vi "GetRelativeAngle.vi"(8 "error in (no error)":errorcluster, 10 "Boat Angle":dbl, 11 "Angle in":refnum<class "Angle.lvclass">) -> (0 "error out":errorcluster, 2 "Relative Angle":dbl)   [LabVIEW 2011, in "Angle.lvclass"]
uses:
  Angle.lvclass
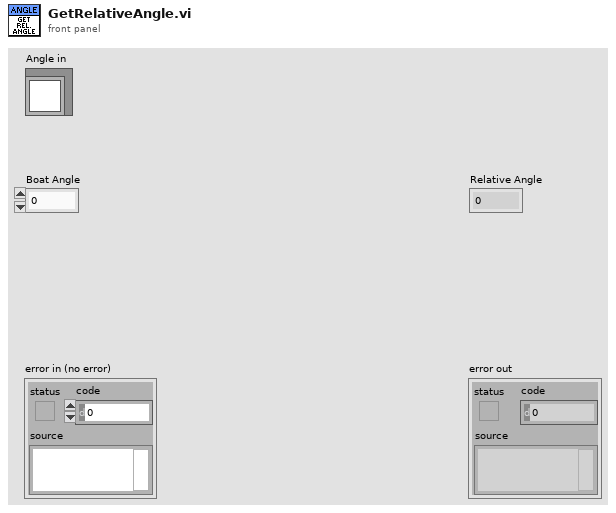
[diagram p1: front panel]
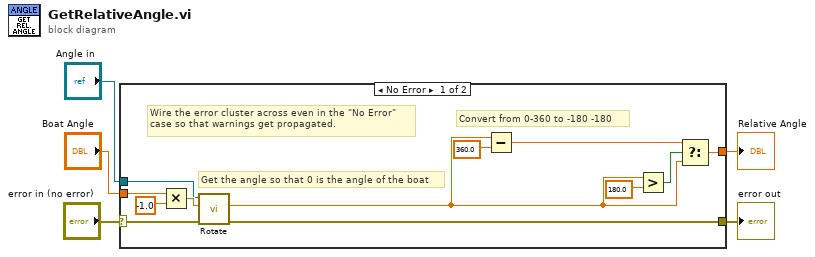
[diagram p0: block diagram]
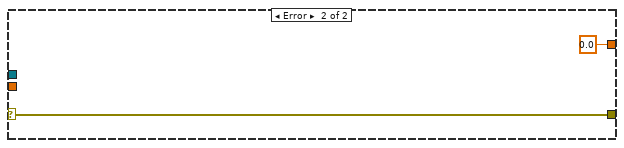
[diagram p2: hidden frame]
diagram:
  n1 = case shown="No Error" "error in (no error)" {
    selector: "error in (no error)" -> [w17 w19]
    tunnel: [w16 w19] -> w4
    tunnel: "Angle in" -> [w12 _]
    tunnel: "Boat Angle" -> [w14 _]
    tunnel: [w6 0.0 ("New Angle")] -> w1
    frame No Error {
      # "Convert from 0-360 to -180 -180"
      # "Get the angle so that 0 is the angle of the boat"
      # "Wire the error cluster across even in the \"No Error\"\ncase so that warnings get propagated."
      n2 = Multiply(x=w14, y=-1.0) -> (x*y=w15:dbl)
      n3 = call "Rotate.vi"("error in (no error)"=w17, "Rotation Angle (Deg.)"=w15, "Angle in"=w12) -> ("error out"=w16:errorcluster, "New Angle"=w7:dbl)  [unwired: 6 in, 1 out]
      n4 = Subtract(x=w7, y=360.0) -> (x-y=w9:dbl)
      n5 = Greater?(x=w7, y=180.0) -> (0:w11:bool)
      n6 = Select(t=w9, s=w11, f=w7) -> (s? t:f=w6:dbl)
    }
    frame Error {
    }
  }
  "error out" <- w4
  "Relative Angle" <- w1
